vi "UTF Time Measurement.vi"() -> (2 "UTF Results":T1[](array[typedef]), 3 "UTF Testing time (seconds)":dbl)   [LabVIEW 2018]
uses:
  <vilib>/utf/common/utf_test_result.ctl
  <vilib>/utf/NI_UnitTestFramework.lvlib
panel:
  out "Project Path":string
  # "UTF"
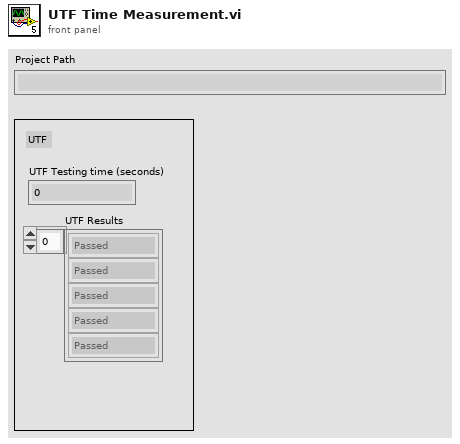
[diagram p1: front panel]
types:
  T1 = typedef "NI_UnitTestFramework.lvlib/utf_test_result.ctl" = enum16{"Passed", "Failed", "Error", "Skipped", "Not Processed"}
  T2 = typedef "NI_UnitTestFramework.lvlib/utf_test_result_overall.ctl" = cluster{"utf results out":T3[], "untested VIs":cluster{"VI path":path, "code coverage":T11, "vi hierarchy":string[]}[], "project file path":path, "system information":string}
  T3 = typedef "NI_UnitTestFramework.lvlib/utf_test_result_testfile.ctl" = cluster{"test case":T4[], "test status":T1, "test path":path, "setup VI":path, "teardown VI":path, "code coverage":T11, "start time":timestamp, "end time":timestamp, "test hierarchy":string[], "VI path":path, "VI timestamp":timestamp, "VI rev hist":i32, "requirements ID":string, "array brackets":string, "name separator":string, "errors":T12[], "paragraph header":string, "result comment":string, "vi hierarchy":string[], "subVI coverage info":T11[], "subVI info":T14[], "big array threshold":u32, "VI Index":i32, "Comment":string, "Dynamic Dispatch":bool, "User-defined test VI":path, "user-defined VI code coverage":T11}
  T4 = typedef "NI_UnitTestFramework.lvlib/utf_test_result_testcase.ctl" = cluster{"test result":T1, "run Times":T5[], "test case name":string, "requirements":string, "code coverage":T11, "subVI coverage info":T11[]}
  T5 = typedef "NI_UnitTestFramework.lvlib/utf_test_result_troll_new.ctl" = cluster{"result (test)":T1, "Vector Result":T6[]}
  T6 = typedef "NI_UnitTestFramework.lvlib/utf_vector_result.ctl" = cluster{"time elapsed [ms]":u32, "result (test)":T1, "result (parameters)":T7[], "Used Vector Values":cluster{"Vector Name":string, "element":i32}[], "Executed Class Path":path, "Input":T10[]}
  T7 = typedef "NI_UnitTestFramework.lvlib/utf_test_result_failure.ctl" = cluster{"result":T1, "error message":string, "parameter name":string, "parameter value":variant, "parameters":variant[], "comparison":T8, "requirement ID":string, "VI":T9, "Used Vector Name":string}
  T8 = typedef "NI_UnitTestFramework.lvlib/utf_test_comparison_operators.ctl" = enum16{"=", "!=", ">", ">=", "<", "<=", "range", "symmetric tolerance", "asymmetric tolerance", "string contains", "string not contain", "array size", "string length", "array range", "by element", "array range (limit array)", "user-defined", "array contains", "array not contain", "vector length", "= (elm)", "!= (elm)", "= (case insensitive)", "!= (case insensitive)"}
  T9 = typedef "NI_UnitTestFramework.lvlib/utf_vi_tag.ctl" = enum16{"Setup VI", "VI under Test", "Teardown VI"}
  T10 = typedef "NI_UnitTestFramework.lvlib/utf_test_result_input_data.ctl" = cluster{"Name":string, "Input Value":variant[], "VI":T9, "Used Vector Index":i32}
  T11 = typedef "NI_UnitTestFramework.lvlib/utf_code_coverage.ctl" = cluster{"coverage":dbl, "diagram run flag":bool[]}
  T12 = typedef "NI_UnitTestFramework.lvlib/utf_error_data.ctl" = cluster{"error type":T13, "description":string}
  T13 = typedef "NI_UnitTestFramework.lvlib/utf_error_type.ctl" = enum16{"TestFileError", "VIError", "SetupVIError", "TearDownVIError", "OtherError"}
  T14 = typedef "NI_UnitTestFramework.lvlib/utf_subvi_info.ctl" = cluster{"Path":path, "Dependence VI":bool}
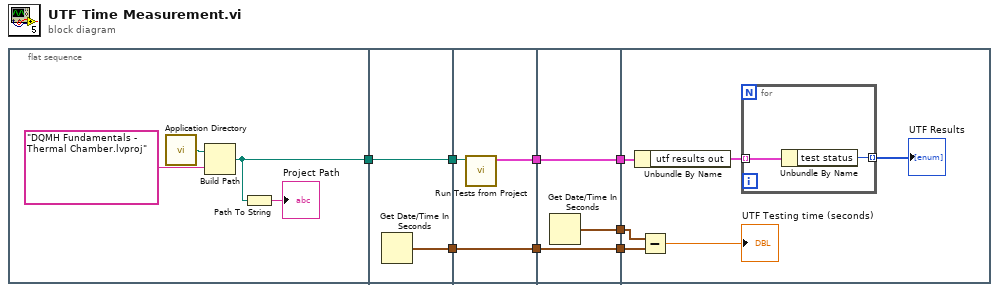
[diagram p0: block diagram]
diagram:
  n1 = flat-sequence {
    tunnel: [w10] -> w1
    tunnel: [w14] -> w8
    tunnel: [w13] -> w2
    tunnel: w1 -> [w13]
    tunnel: [w17] -> w7
    tunnel: w8 -> [w17]
    tunnel: [w16] -> w3
    tunnel: w2 -> [w15]
    tunnel: [w20] -> w6
    tunnel: [w19] -> w5
    tunnel: w7 -> [w19]
    tunnel: [w18] -> w4
    tunnel: w3 -> [w18]
    tunnel: w6 -> [w25]
    tunnel: w5 -> [w26]
    tunnel: w4 -> [w22]
    frame #0 {
      n2 = call <vilib>:"Application Directory.vi"() -> ("Application Directory"=w9:path)
      n3 = Build Path(base path=w9, name or relative path="DQMH Fundamentals - Thermal Chamber.lvproj" ("Project Name")) -> (appended path=w10:path)
      n4 = Path To String(path=w10) -> (string=→"Project Path":string)
    }
    frame #1 {
      n5 = Get Date/Time In Seconds() -> (seconds since 1Jan1904=w14:timestamp)
    }
    frame #2 {
      n6 = call <vilib>:"Run Tests from Project.vi"("project file path"=w15) -> ("test results out"=w16:T2)  [unwired: 9 in, 1 out]
    }
    frame #3 {
      n7 = Get Date/Time In Seconds() -> (seconds since 1Jan1904=w20:timestamp)
    }
    frame #4 {
      n8 = Unbundle By Name(w22) -> ("utf results out"=w23:T3[])
      n9 = Subtract(x=w25, y=w26) -> (x-y=→"UTF Testing time (seconds)":dbl)
      n10 = for {
        tunnel: [w28] -> w24 mode=indexing
        tunnel: w23 -> [w27] mode=indexing
        n11 = Unbundle By Name(w27) -> ("test status"=w28:T1)
      }
      "UTF Results" <- w24
    }
  }
